vi "Modified Measuring Y verses V(1).vi"() -> ()   [LabVIEW 2020]
uses:
  <vilib>/DAQmx/write.llb/DAQmx Write (Analog 1D DBL 1Chan NSamp).vi
  <vilib>/DAQmx/create/channels.llb/DAQmx Create Channel (AO-Voltage-Basic).vi
  <vilib>/DAQmx/configure/timing.llb/DAQmx Timing (Sample Clock).vi
  <vilib>/Utility/file.llb/Read Delimited Spreadsheet (DBL).vi
  <vilib>/DAQmx/miscellaneous.llb/DAQmx Fill In Error Info.vi
  <vilib>/DAQmx/create/channels.llb/DAQmx Create Channel (CO-Pulse Generation-Frequency).vi
  <vilib>/DAQmx/configure/timing.llb/DAQmx Timing (Implicit).vi
  <resource>/objmgr/daqmx.rc
panel:
  in  "Number of datapoints":i32=100
  in  "File to read":path=path "C:/Users/Hannah/Downloads/50mmcl_calibration_100points_transposed.txt"
  out "actual frequency":dbl=1.0
  in  "stop":bool
  out "Signal input to voice coil (blue)":dbl[](graph)=[-0.25, -0.245, -0.24, -0.235, -0.23, -0.225, -0.22, -0.215, -0.211, -0.206, -0.201, -0.196, -0.191, -0.186, -0.181, -0.176, -0.171, -0.166, -0.161, -0.156, -0.151, -0.146, -0.142, -0.137, -0.132, -0.127, -0.122, -0.117, -0.112, -0.107, -0.102, -0.097, -0.092, -0.087, -0.082, -0.077, -0.073, -0.068, -0.063, -0.058, -0.053, -0.048, -0.043, -0.038, -0.033, -0.028, -0.023, -0.018, -0.013, -0.008, -0.004, 0.001, 0.006, 0.011, 0.016, 0.021, 0.026, 0.031, 0.036, 0.041, 0.046, 0.051, 0.056, 0.061, 0.065, 0.07, 0.075, 0.08, 0.085, 0.09, 0.095, 0.1, 0.105, 0.11, 0.115, 0.12, 0.125, 0.13, 0.134, 0.139, 0.144, 0.149, 0.154, 0.159, 0.164, 0.169, 0.174, 0.179, 0.184, 0.189, 0.194, 0.199, 0.203, 0.208, 0.213, 0.218, 0.223, 0.228, 0.233, 0.238]
  out "# Samples written per channel":u32=100
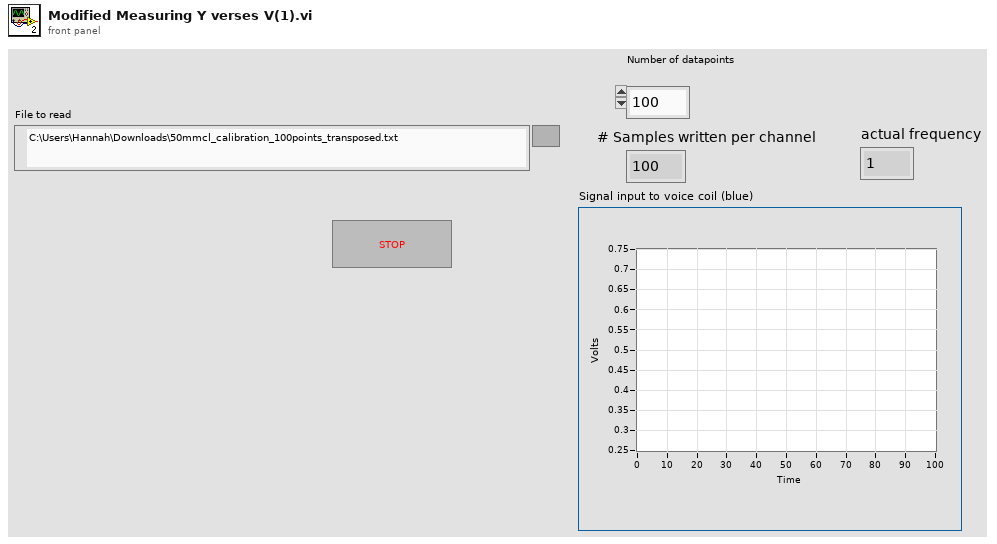
[diagram p1: front panel]
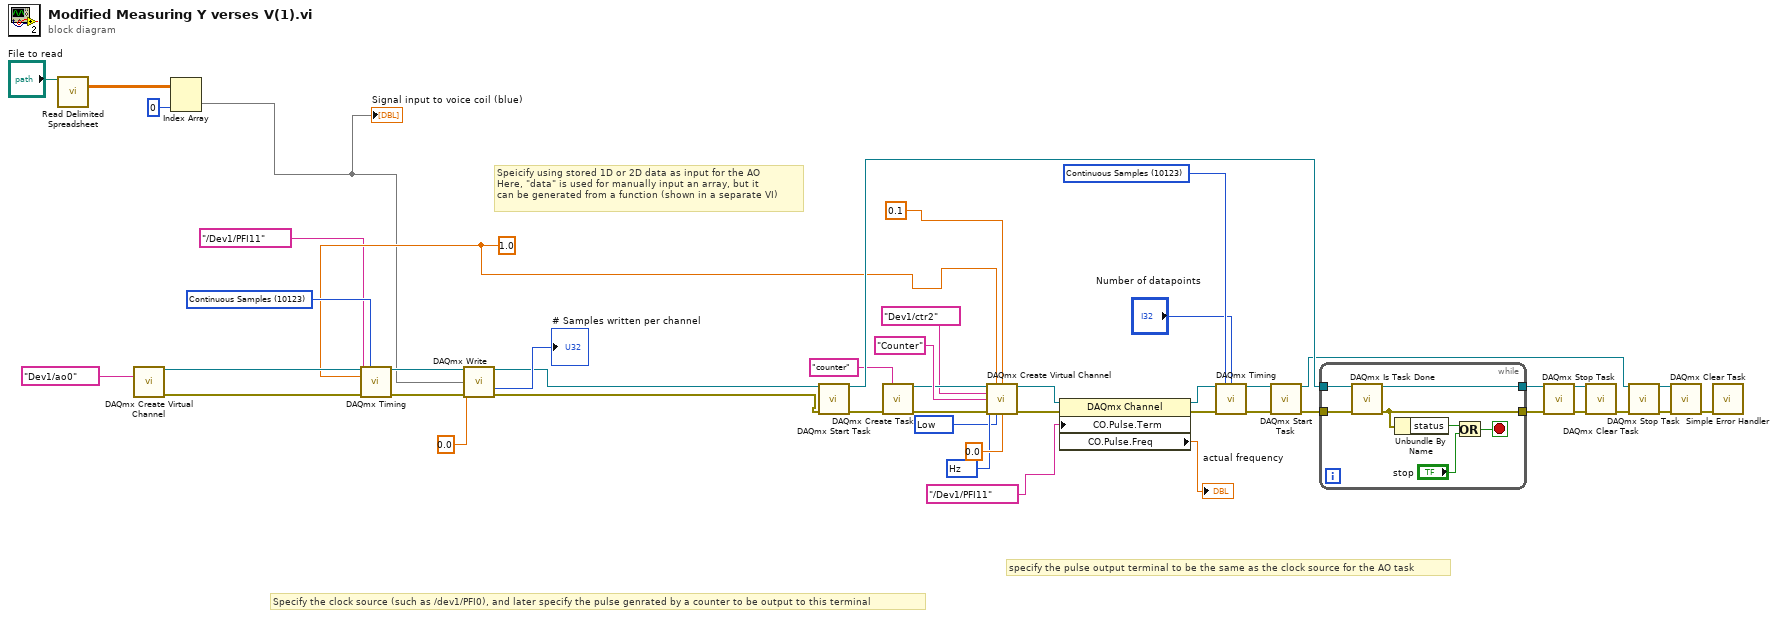
[diagram p0: block diagram]
diagram:
  w9 = 10214 items=["High"=10192, "Low"=10214] ("idle state")
  w10 = 10373 items=["Hz"=10373] ("units")
  w39 = 10123 items=["Finite Samples"=10178, "Continuous Samples"=10123, "Hardware Timed Single Point"=12522] ("sample mode")
  w7 = 1.0 ("rate")
  w45 = 10123 items=["Finite Samples"=10178, "Continuous Samples"=10123, "Hardware Timed Single Point"=12522] ("sample mode")
  # "specify the pulse output terminal to be the same as the clock source for the AO task"
  # "Speicify using stored 1D or 2D data as input for the AO\nHere, \"data\" is used for manually input an array, but it\ncan be generated from a function (shown in a separate VI)"
  # "Specify the clock source (such as /dev1/PFI0), and later specify the pulse genrated by a counter to be output to this terminal"
  n1 = call-poly <vilib>:"Read Delimited Spreadsheet.vi"("file path (dialog if empty)"="File to read") -> ("all rows"=w4:dbl[][])  [unwired: 9 in, 5 out]
  n2 = call-poly <vilib>:"DAQmx Create Virtual Channel.vi"("physical channels"=tag "Dev1/ao0") -> ("task out"=w47:refnum<k21>, "error out"=w46:errorcluster)  [unwired: 13 in]
  n3 = Index Array(array=w4, index (col)=0 ("disabled index (col)")) -> (element=w2:dbl[])  [unwired: 1 in]
  "Signal input to voice coil (blue)" <- w2
  n4 = call-poly <vilib>:"DAQmx Timing.vi"("task/channels in"=w47, "sample mode"=w45, "rate"=w7, "source"=tag "/Dev1/PFI11", "error in"=w46) -> ("task out"=w41:refnum<k21>, "error out"=w44:errorcluster)  [unwired: 9 in]
  n5 = call-poly <vilib>:"DAQmx Write.vi"("task/channels in"=w41, "data"=w2, "timeout"=0.0, "error in"=w44) -> ("task out"=w16:refnum<k21>, "number of samples written per channel"=→"# Samples written per channel":u32, "error out"=w15:errorcluster)  [unwired: 9 in]
  n6 = call <vilib>:"DAQmx Start Task.vi"("task/channels in"=w16, "error in"=w15) -> ("task out"=w40:refnum<k21>, "error out"=w18:errorcluster)  [unwired: 12 in]
  n7 = call <vilib>:"DAQmx Create Task.vi"("new task name"="counter", "error in"=w18) -> ("task out"=w35:refnum<k21>, "error out"=w33:errorcluster)  [unwired: 12 in]
  n8 = call-poly <vilib>:"DAQmx Create Virtual Channel.vi"("task in"=w35, "frequency"=w7, "duty cycle"=0.1, "counter"=tag "Dev1/ctr2", "name to assign"="Counter", "units"=w10, "error in"=w33, "idle state"=w9, "initial delay"=0.0) -> ("task out"=w32:refnum<k21>, "error out"=w31:errorcluster)  [unwired: 5 in]
  n9 = property class="DAQmx Channel"(reference=w32, error in=w31, "CO.Pulse.Term"=tag "/Dev1/PFI11") -> (reference out=w28:refnum<k21>, error out=w29:errorcluster, "CO.Pulse.Freq"=→"actual frequency":dbl)
  n10 = call-poly <vilib>:"DAQmx Timing.vi"("task/channels in"=w28, "sample mode"=w39, "samples per channel"="Number of datapoints", "error in"=w29) -> ("task out"=w38:refnum<k21>, "error out"=w37:errorcluster)  [unwired: 10 in]
  n11 = call <vilib>:"DAQmx Start Task.vi"("task/channels in"=w38, "error in"=w37) -> ("task out"=w27:refnum<k21>, "error out"=w17:errorcluster)  [unwired: 12 in]
  n12 = while {
    tunnel: w40 -> [w54]
    tunnel: w17 -> [w53]
    tunnel: [w52] -> w23
    tunnel: [w51] -> w24
    stop <- w48 stop-if-true
    n13 = call <vilib>:"DAQmx Is Task Done.vi"("task/channels in"=w54, "error in"=w53) -> ("task out"=w52:refnum<k21>, "error out"=w51:errorcluster)  [unwired: 11 in, 1 out]
    n14 = Unbundle By Name(w51) -> ("status"=w50:bool)
    n15 = Or(x=w50, y="stop") -> (x .or. y?=w48:bool)
  }
  n16 = call <vilib>:"DAQmx Stop Task.vi"("task/channels in"=w23, "error in"=w24) -> ("task out"=w22:refnum<k21>, "error out"=w21:errorcluster)  [unwired: 12 in]
  n17 = call <vilib>:"DAQmx Clear Task.vi"("task in"=w22, "error in"=w21) -> ("error out"=w20:errorcluster)  [unwired: 13 in]
  n18 = call <vilib>:"DAQmx Stop Task.vi"("task/channels in"=w27, "error in"=w20) -> ("task out"=w25:refnum<k21>, "error out"=w26:errorcluster)  [unwired: 12 in]
  n19 = call <vilib>:"DAQmx Clear Task.vi"("task in"=w25, "error in"=w26) -> ("error out"=w19:errorcluster)  [unwired: 13 in]
  n20 = call <vilib>:"Simple Error Handler.vi"("error in (no error)"=w19) -> ()  [unwired: 4 in, 5 out]
